vi "Untitled.vi"() -> ()   [LabVIEW 2020]
panel:
  in  "path to BMP file":path
  out "new picture 2":picture
  in  "8-bit pixmap":u8[][](array[numeric])
  out "new picture":picture
  in  "colors":u32[](array[numeric])
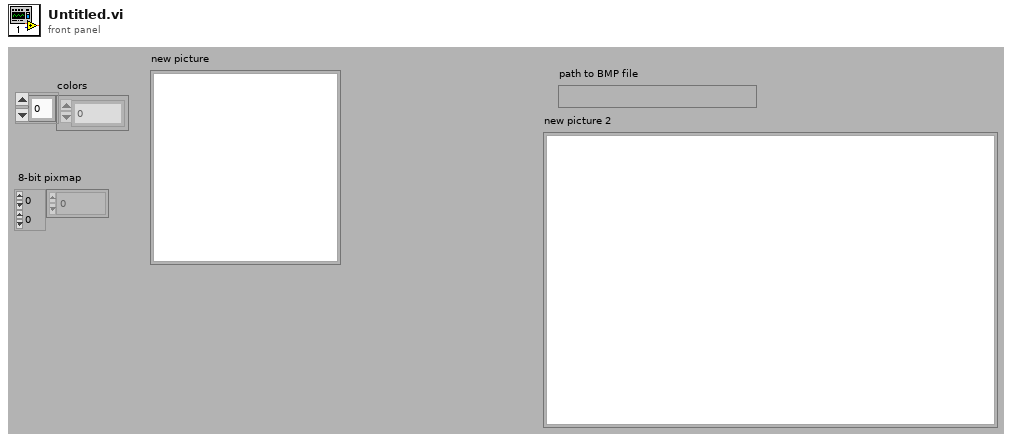
[diagram p1: front panel]
types:
  T1 = typedef "imagedata.ctl" = cluster{"image type":i32, "image depth":i32, "image":u8[], "mask":u8[], "colors":u32[], "Rectangle":cluster{"left":i16, "top":i16, "right":i16, "bottom":i16}}
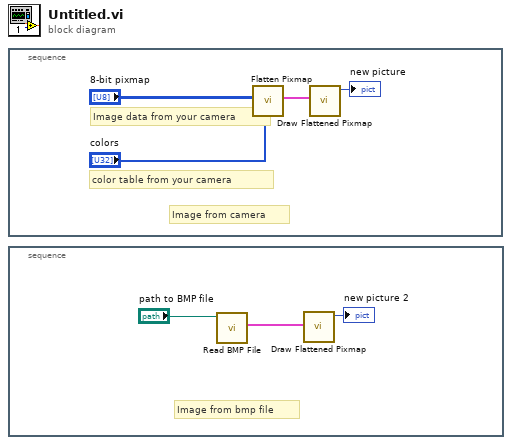
[diagram p0: block diagram]
diagram:
  n1 = stacked-sequence {
    frame #0 {
      # "Image from camera"
      # "Image data from your camera"
      # "color table from your camera"
      n2 = call <vilib>:"Flatten Pixmap.vi"("colors"="colors", "8-bit pixmap"="8-bit pixmap") -> ("image data"=w4:T1)  [unwired: 9 in]
      n3 = call <vilib>:"Draw Flattened Pixmap.vi"("image data"=w4) -> ("new picture"=→"new picture":picture)  [unwired: 8 in]
    }
  }
  n4 = stacked-sequence {
    frame #0 {
      # "Image from bmp file"
      n5 = call <vilib>:"Read BMP File.vi"("path to BMP file"="path to BMP file") -> ("image data"=w7:T1)  [unwired: 8 in, 2 out]
      n6 = call <vilib>:"Draw Flattened Pixmap.vi"("image data"=w7) -> ("new picture"=→"new picture 2":picture)  [unwired: 8 in]
    }
  }
